vi "AO_mini_AndorEMCCD.vi"() -> ()   [LabVIEW 2018]
panel:
  in  "Auto Scale":bool=TRUE caption="PD Correction"
  out "Get EMCCD Gain":i32=1
  in  "Spool":bool=TRUE caption="Cameras Live Display"
  out "Return from SetSpool":i32=1
  out "Running Status":T1(ring) caption="Camera FOV"
  out "Return from Start Acquisition":u32
  out "Return from GetAcquiredData":u32
  in  "Folder Name":string="test"
  in  "File Type":enum16{"TIFF", "Sif"}(ring)
  out "Return from CheckProcess":u32
  out "Get Kinetic Time":sgl format="%.4f"
  out "Get Accum Time":sgl format="%.4f"
  out "Get Kinetic Num":i32=1
  out "Get Accum Num":i32=1
  in  "Abort":bool
  out "FOV Y Pixels":i32
  out "FOV X Pixels":i32
  in  "Acquisition":bool
  in  "Exit":bool
  out "EMCCD Status":bool
  in  "Stop LIVE":bool
  in  "Start LIVE":bool
  out "error out":errorcluster
  out "Return from CheckTimings":u32
  out "Get Exposure Time":sgl format="%.4f"
  in  "error in (no error)":errorcluster
  in  "Intensity Min":dbl=200.0 min=1.0
  in  "Intensity Max":dbl=10000.0 min=1.0
  in  "Shutdown EMCCD when exit":bool=TRUE caption="PD Correction"
  in  "Update FOV":bool
  in  "Update AcqSetting":bool
  in  "Exposure time (s)":dbl=0.02
  in  "Main Path":path=path "D:/Data"
  in  "File Name":string="test"
  in  "Kinetic Num":u32=5
  in  "Accum Num":u32=2
  in  "Initialize EMCCD":bool=TRUE caption="PD Correction"
  in  "CoolToTargetTemp":bool=TRUE caption="PD Correction"
  out "Intensity Graph":i32[][](graph)
  out "Current Temp":i32
  out "Detector Y Pixels":i32
  out "Detector X Pixels":i32
  in  "Aquisition Mode":T2(ring)=enum."Single Scan" caption="Camera FOV"
  in  "Trigger Mode":enum16{"Internal", "External"}(ring) caption="Camera FOV"
  in  "Gain Value":sgl=20.0 format="%.2f"
  in  "Yend":i32=1002
  in  "Xend":i32=1004
  in  "Ystart":i32=2
  in  "Xstart":i32=2
  in  "Ybin":i32=1
  in  "Xbin":i32=1
  in  "Camera FOV":T3(ring)=enum."Full FOV"
  in  "Gain On":bool=TRUE caption="Cameras Live Display"
  in  "Set Temp":i32=-60
  # "It takes some time to warm up / cool down the camera when initializing or shuting down the camera (without Temp feedback)"
  # "C"
  # "Acquisition Settings"
  # "Status"
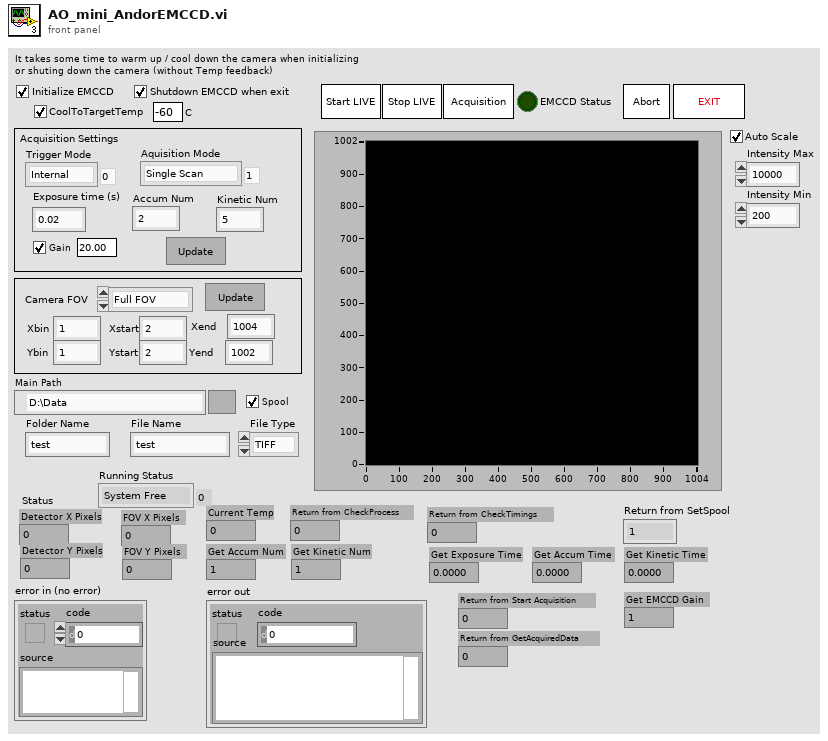
[diagram p1: front panel]
types:
  T1 = enum16{"System Free", "Live Preview", "Data Acquisition"}
  T2 = enum16{"None", "Single Scan", "Accumulate", "Kinetics", "Fast Kinetics", "Run till abort"}
  T3 = enum16{"Custom FOV", "Full FOV", "FOV: 768x768", "FOV: 512x512", "FOV: 320x320", "FOV: 256x256", ""}
  T4 = typedef "Error Code Enum typedef.ctl" = enum32{"N/A (0)", "DRV_ERROR_CODES", "DRV_SUCCESS", "DRV_VXDNOTINSTALLED", "DRV_ERROR_SCAN", "DRV_ERROR_CHECK_SUM", "DRV_ERROR_FILELOAD", "DRV_UNKNOWN_FUNC", "DRV_ERROR_VXD_INIT", "DRV_ERROR_ADDRESS", "DRV_ERROR_PAGELOCK", "DRV_ERROR_PAGEUNLOCK", "DRV_ERROR_BOARDTEST", "DRV_ERROR_ACK", "DRV_ERROR_UP_FIFO", "DRV_ERROR_PATTERN", "N/A (16)", "DRV_ACQUISITION_ERRORS", "DRV_ACQ_BUFFER", "DRV_ACQ_DOWNFIFO_FULL", "DRV_PROC_UNKONWN_INSTRUCTION", "DRV_ILLEGAL_OP_CODE", "DRV_KINETIC_TIME_NOT_MET", "DRV_ACCUM_TIME_NOT_MET", "DRV_NO_NEW_DATA", "N/A (25)", "DRV_SPOOLERROR", "N/A (27)", "N/A (28)", "N/A (29)", "N/A (30)", "N/A (31)", "N/A (32)", "DRV_TEMPERATURE_CODES", "DRV_TEMPERATURE_OFF", "DRV_TEMPERATURE_NOT_STABILIZED", "DRV_TEMPERATURE_STABILIZED", "DRV_TEMPERATURE_NOT_REACHED", "DRV_TEMPERATURE_OUT_RANGE", "DRV_TEMPERATURE_NOT_SUPPORTED", "DRV_TEMPERATURE_DRIFT", "N/A (41)", "N/A (42)", "N/A (43)", "N/A (44)", "N/A (45)", "N/A (46)", "N/A (47)", "N/A (48)", "DRV_GENERAL_ERRORS", "DRV_INVALID_AUX", "DRV_COF_NOTLOADED", "DRV_FPGAPROG", "DRV_FLEXERROR", "DRV_GPIBERROR", "N/A (55)", "N/A (56)", "N/A (57)", "N/A (58)", "N/A (59)", "N/A (60)", "N/A (61)", "N/A (62)", "N/A (63)", "DRV_DATATYPE", "DRV_DRIVER_ERRORS", "DRV_P1INVALID", "DRV_P2INVALID", "DRV_P3INVALID", "DRV_P4INVALID", "DRV_INIERROR", "DRV_COFERROR", "DRV_ACQUIRING", "DRV_IDLE", "DRV_TEMPCYCLE", "DRV_NOT_INITIALIZED", "DRV_P5INVALID", "DRV_P6INVALID", "DRV_INVALID_MODE", "DRV_INVALID_FILTER", "DRV_I2CERRORS", "DRV_I2CDEVNOTFOUND", "DRV_I2CTIMEOUT", "DRV_P7INVALID", "N/A (84)", "N/A (85)", "N/A (86)", "N/A (87)", "N/A (88)", "N/A (89)", "DRV_IOCERROR", "DRV_VRMVERSIONERROR"}
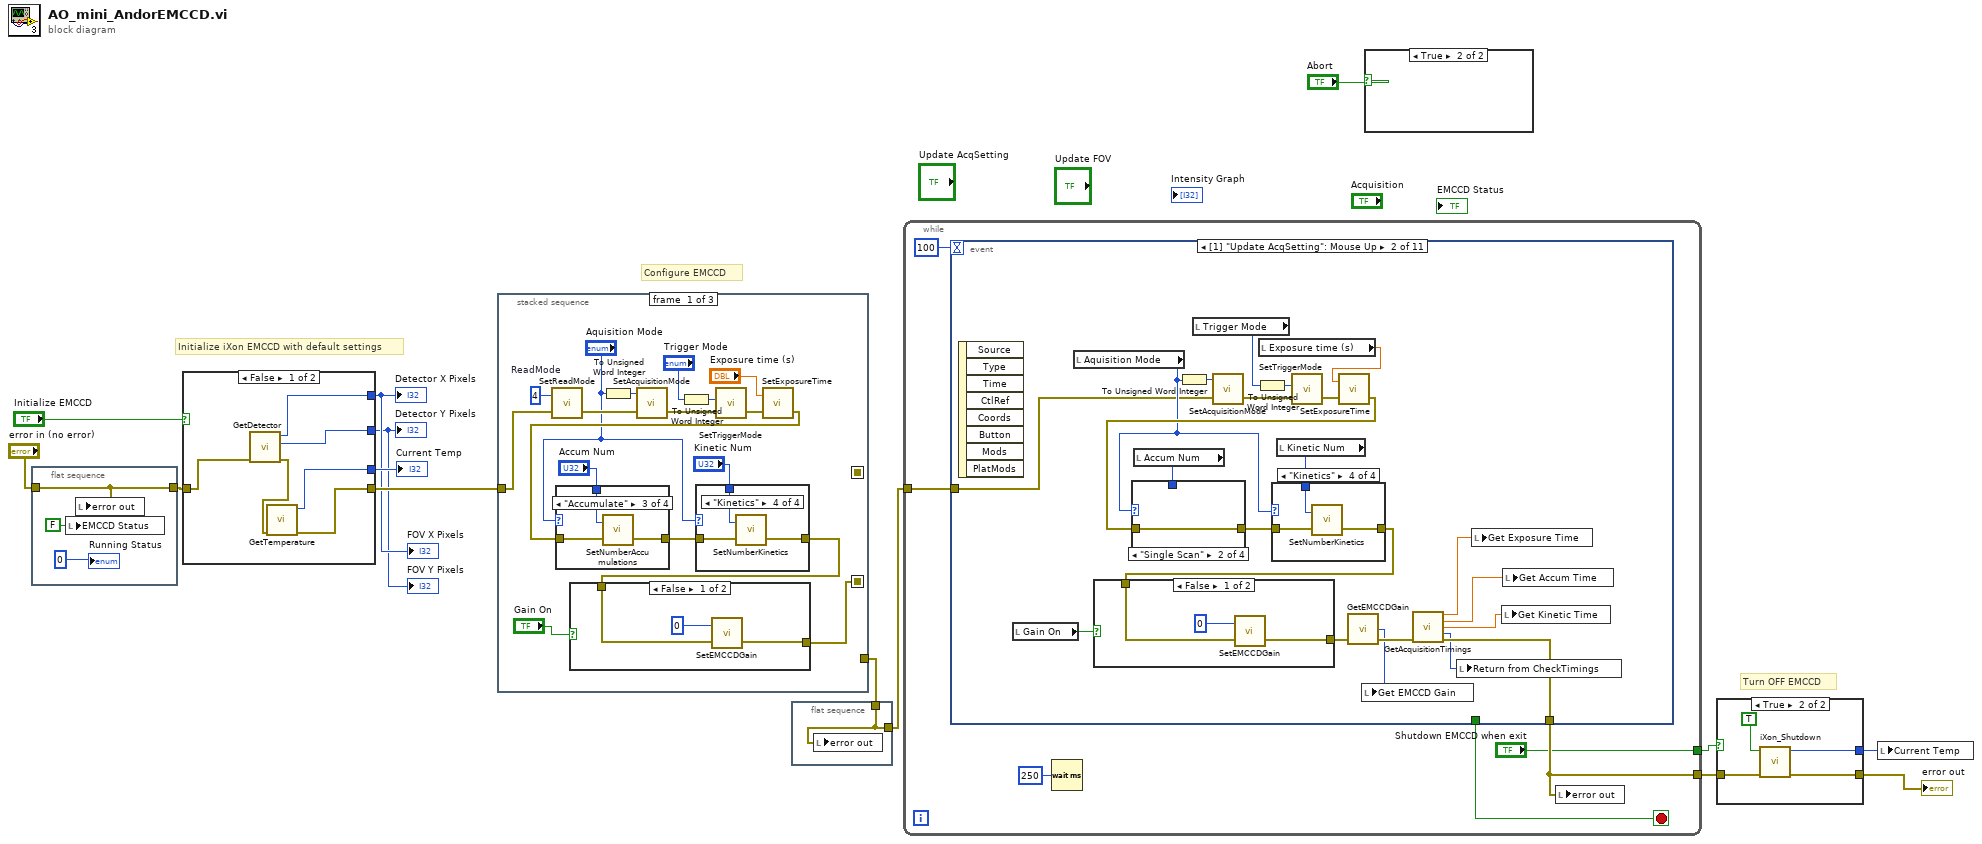
[diagram p0: block diagram]
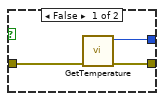
[diagram p3: hidden frame]
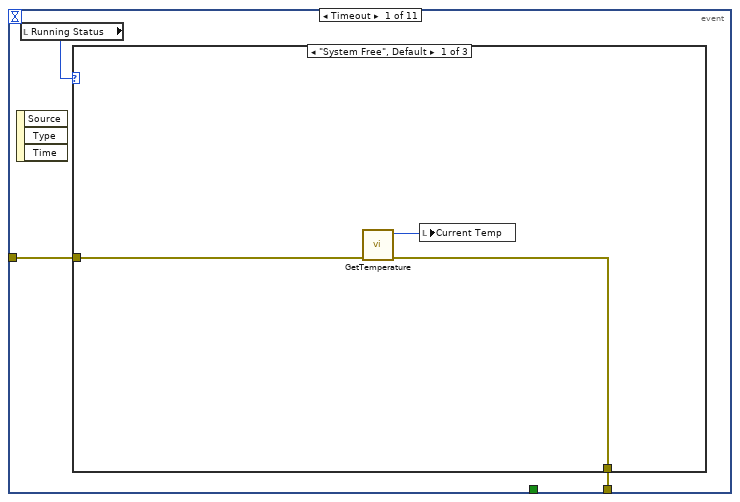
[diagram p4: hidden frame]
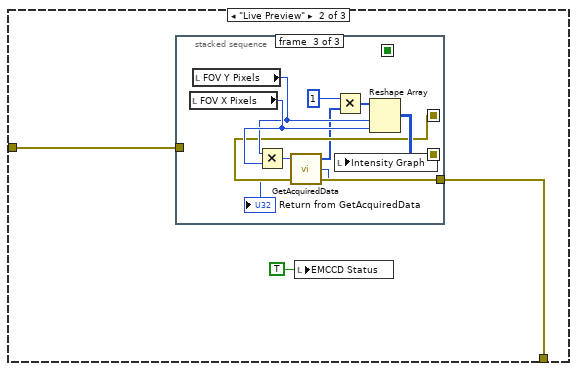
[diagram p5: hidden frame]
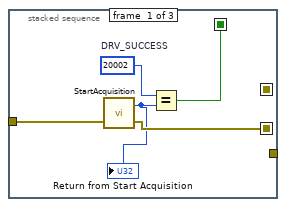
[diagram p6: hidden frame]
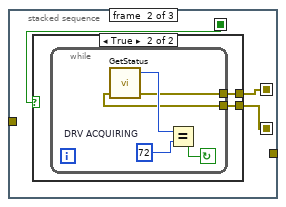
[diagram p7: hidden frame]
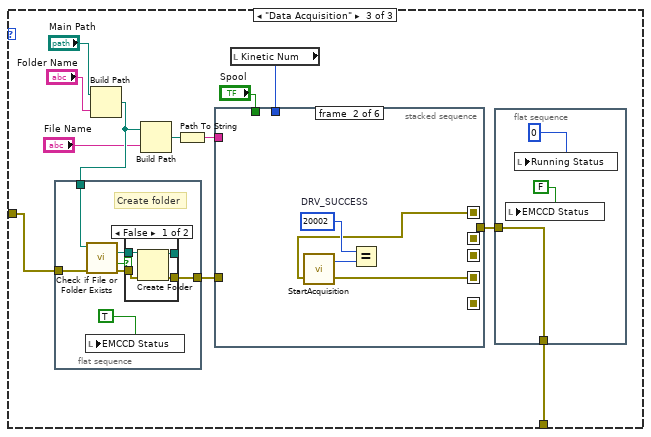
[diagram p9: hidden frame]
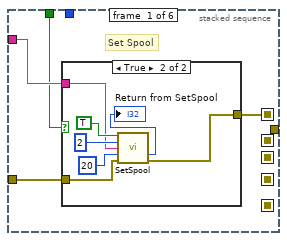
[diagram p10: hidden frame]
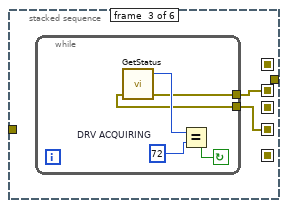
[diagram p12: hidden frame]
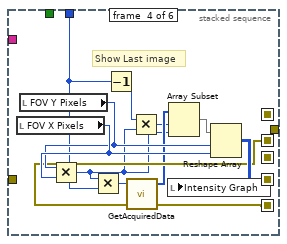
[diagram p13: hidden frame]
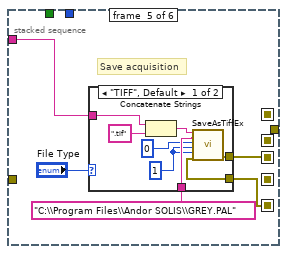
[diagram p14: hidden frame]
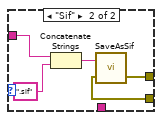
[diagram p15: hidden frame]
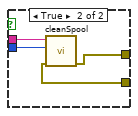
[diagram p17: hidden frame]
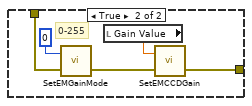
[diagram p19: hidden frame]
diagram:
  # "Turn OFF EMCCD"
  # "Configure EMCCD"
  # "Initialize iXon EMCCD with default settings"
  n1 = flat-sequence {
    tunnel: "error in (no error)" -> [w17]
    tunnel: [w17] -> w5
    frame #0 {
      n2 = local write "EMCCD Status"(FALSE) -> ()
      n3 = local write "error out"(w17) -> ()
      "Running Status" <- u16 0
    }
  }
  n4 = case shown="False" "Initialize EMCCD" {
    tunnel: w5 -> [w22 w29]
    tunnel: [w20 w27] -> w11
    tunnel: [w19 w26] -> w10
    tunnel: [w23 w25] -> w13
    tunnel: [w18 w24] -> w12
    frame False {
      n5 = call <userlib>:"GetDetector.vi"("error in (no error)"=w22) -> ("error out"=w21:errorcluster, "ypixels"=w19:i32, "xpixels"=w20:i32)  [unwired: 3 in, 1 out]
      n6 = call <userlib>:"GetTemperature.vi"("error in (no error)"=w21) -> ("error out"=w18:errorcluster, "temperature"=w23:i32)  [unwired: 3 in, 2 out]
    }
    frame True {
      n7 = call "iXon_Init_Cool.vi"("error in (no error)"=w29, "CoolToTargetTemp"="CoolToTargetTemp", "Set Temp"="Set Temp") -> ("error out"=w24:errorcluster, "Current Temp"=w25:i32, "Detector Y Pixels"=w26:i32, "Detector X Pixels"=w27:i32)  [unwired: 5 in]
    }
  }
  "Detector X Pixels" <- w11
  "Detector Y Pixels" <- w10
  "Current Temp" <- w13
  "FOV X Pixels" <- w11
  "FOV Y Pixels" <- w10
  n8 = stacked-sequence {
    seq-local: [w31 _ _] -> [_ w75 _]
    seq-local: [_ w74 _] -> [_ _ w173]
    tunnel: w12 -> [w45 _ _]
    tunnel: [_ _ w165] -> w4
    frame #0 {
      w46 = u16 4  # ReadMode
      n9 = call <userlib>:"SetReadMode.vi"("error in (no error)"=w45, "mode"=w46) -> ("error out"=w43:errorcluster)  [unwired: 1 out]
      n10 = To Unsigned Word Integer(number="Aquisition Mode") -> (unsigned 16bit integer=w47:u16)
      n11 = call <userlib>:"SetAcquisitionMode.vi"("error in (no error)"=w43, "mode"=w47) -> ("error out"=w42:errorcluster)  [unwired: 1 out]
      n12 = To Unsigned Word Integer(number="Trigger Mode") -> (unsigned 16bit integer=w41:u16)
      n13 = call <userlib>:"SetTriggerMode.vi"("error in (no error)"=w42, "mode"=w41) -> ("error out"=w40:errorcluster)  [unwired: 1 out]
      n14 = call <userlib>:"SetExposureTime.vi"("error in (no error)"=w40, "time"="Exposure time (s)") -> ("error out"=w37:errorcluster)  [unwired: 1 out]
      n15 = case shown="\"Accumulate\"" "Aquisition Mode" {
        tunnel: "Accum Num" -> [_ _ w66 w69]
        tunnel: w37 -> [w62 w63 w65 w68]
        tunnel: [w62 w63 w64 w67] -> w36
        frame "None", Default {
        }
        frame "Single Scan" {
        }
        frame "Accumulate" {
          n16 = call <userlib>:"SetNumberAccumulations.vi"("error in (no error)"=w65, "number"=w66) -> ("error out"=w64:errorcluster)  [unwired: 1 out]
        }
        frame "Kinetics" {
          n17 = call <userlib>:"SetNumberAccumulations.vi"("error in (no error)"=w68, "number"=w69) -> ("error out"=w67:errorcluster)  [unwired: 1 out]
        }
      }
      n18 = case shown="\"Kinetics\"" "Aquisition Mode" {
        tunnel: w36 -> [w56 w57 w58 w61]
        tunnel: [w56 w57 w58 w60] -> w32
        tunnel: "Kinetic Num" -> [_ _ _ w59]
        frame "None", Default {
        }
        frame "Single Scan" {
        }
        frame "Accumulate" {
        }
        frame "Kinetics" {
          n19 = call <userlib>:"SetNumberKinetics.vi"("error in (no error)"=w61, "number"=w59) -> ("error out"=w60:errorcluster)  [unwired: 1 out]
        }
      }
      n20 = case shown="False" "Gain On" {
        tunnel: w32 -> [w50 w55]
        tunnel: [w49 w52] -> w31
        frame False {
          n21 = call <userlib>:"SetEMCCDGain.vi"("error in (no error)"=w50, "gain"=u16 0) -> ("error out"=w49:errorcluster)  [unwired: 1 out]
        }
        frame True {
          # "0-255"
          n22 = call <userlib>:"SetEMGainMode.vi"("error in (no error)"=w55, "mode"=0) -> ("error out"=w53:errorcluster)  [unwired: 1 out]
          n23 = call <userlib>:"SetEMCCDGain.vi"("error in (no error)"=w53, "gain"="Gain Value") -> ("error out"=w52:errorcluster)  [unwired: 1 out]
        }
      }
    }
    frame #1 {
      # "Set FOV"
      n24 = local read "Detector X Pixels"() -> (w73:i32)
      n25 = local read "Detector Y Pixels"() -> (w72:i32)
      n26 = case shown="\"Custom FOV\"" "Camera FOV" {
        tunnel: ["Xbin" w112 w128 w144 w160 w163] -> w81
        tunnel: ["Ybin" w112 w128 w144 w160 w163] -> w80
        tunnel: ["Xstart" w102 w118 w134 w150 w163] -> w79
        tunnel: ["Xend" w99 w115 w131 w147 w161] -> w78
        tunnel: ["Ystart" w101 w117 w133 w149 w163] -> w77
        tunnel: ["Yend" w98 w114 w130 w146 w162] -> w76
        tunnel: w73 -> [_ w111 w127 w143 w159 w161]
        tunnel: w72 -> [_ w110 w126 w142 w158 w162]
        tunnel: [w83 w97 w113 w129 w145 w162] -> w71
        tunnel: [w86 w97 w113 w129 w145 w161] -> w70
        frame "Custom FOV" {
          n27 = Subtract(x="Yend", y="Ystart") -> (x-y=w93:i32)
          n28 = Subtract(x="Xend", y="Xstart") -> (x-y=w96:i32)
          n29 = Increment(x=w93) -> (x+1=w90:i32)
          n30 = Increment(x=w96) -> (x+1=w89:i32)
          n31 = Divide(x=w90, y="Ybin") -> (x/y=w84:dbl)
          n32 = Divide(x=w89, y="Xbin") -> (x/y=w87:dbl)
          n33 = To Long Integer(number=w84) -> (32bit integer=w83:i32)
          n34 = To Long Integer(number=w87) -> (32bit integer=w86:i32)
        }
        frame "FOV: 768x768" {
          w97 = 768
          w107 = 2.0
          w112 = 1
          n35 = Subtract(x=w111, y=w97) -> (x-y=w109:i32)
          n36 = Subtract(x=w110, y=w97) -> (x-y=w108:i32)
          n37 = Divide(x=w108, y=w107) -> (x/y=w105:dbl)
          n38 = Divide(x=w109, y=w107) -> (x/y=w106:dbl)
          n39 = Decrement(x=w97) -> (x-1=w100:i32)
          n40 = Round To Nearest(number=w106) -> (nearest integer value=w104:dbl)
          n41 = Round To Nearest(number=w105) -> (nearest integer value=w103:dbl)
          n42 = To Long Integer(number=w104) -> (32bit integer=w102:i32)
          n43 = To Long Integer(number=w103) -> (32bit integer=w101:i32)
          n44 = Add(x=w100, y=w102) -> (x+y=w99:i32)
          n45 = Add(x=w100, y=w101) -> (x+y=w98:i32)
        }
        frame "FOV: 512x512" {
          w113 = 512
          w123 = 2.0
          w128 = 1
          n46 = Subtract(x=w127, y=w113) -> (x-y=w125:i32)
          n47 = Subtract(x=w126, y=w113) -> (x-y=w124:i32)
          n48 = Divide(x=w124, y=w123) -> (x/y=w121:dbl)
          n49 = Divide(x=w125, y=w123) -> (x/y=w122:dbl)
          n50 = Decrement(x=w113) -> (x-1=w116:i32)
          n51 = Round To Nearest(number=w122) -> (nearest integer value=w120:dbl)
          n52 = Round To Nearest(number=w121) -> (nearest integer value=w119:dbl)
          n53 = To Long Integer(number=w120) -> (32bit integer=w118:i32)
          n54 = To Long Integer(number=w119) -> (32bit integer=w117:i32)
          n55 = Add(x=w116, y=w118) -> (x+y=w115:i32)
          n56 = Add(x=w116, y=w117) -> (x+y=w114:i32)
        }
        frame "FOV: 320x320" {
          w129 = 320
          w139 = 2.0
          w144 = 1
          n57 = Subtract(x=w143, y=w129) -> (x-y=w141:i32)
          n58 = Subtract(x=w142, y=w129) -> (x-y=w140:i32)
          n59 = Divide(x=w140, y=w139) -> (x/y=w137:dbl)
          n60 = Divide(x=w141, y=w139) -> (x/y=w138:dbl)
          n61 = Decrement(x=w129) -> (x-1=w132:i32)
          n62 = Round To Nearest(number=w138) -> (nearest integer value=w136:dbl)
          n63 = Round To Nearest(number=w137) -> (nearest integer value=w135:dbl)
          n64 = To Long Integer(number=w136) -> (32bit integer=w134:i32)
          n65 = To Long Integer(number=w135) -> (32bit integer=w133:i32)
          n66 = Add(x=w132, y=w134) -> (x+y=w131:i32)
          n67 = Add(x=w132, y=w133) -> (x+y=w130:i32)
        }
        frame "FOV: 256x256" {
          w145 = 256
          w155 = 2.0
          w160 = 1
          n68 = Subtract(x=w159, y=w145) -> (x-y=w157:i32)
          n69 = Subtract(x=w158, y=w145) -> (x-y=w156:i32)
          n70 = Divide(x=w156, y=w155) -> (x/y=w153:dbl)
          n71 = Divide(x=w157, y=w155) -> (x/y=w154:dbl)
          n72 = Decrement(x=w145) -> (x-1=w148:i32)
          n73 = Round To Nearest(number=w154) -> (nearest integer value=w152:dbl)
          n74 = Round To Nearest(number=w153) -> (nearest integer value=w151:dbl)
          n75 = To Long Integer(number=w152) -> (32bit integer=w150:i32)
          n76 = To Long Integer(number=w151) -> (32bit integer=w149:i32)
          n77 = Add(x=w148, y=w150) -> (x+y=w147:i32)
          n78 = Add(x=w148, y=w149) -> (x+y=w146:i32)
        }
        frame "Full FOV", Default {
          w163 = 1
        }
      }
      n79 = local write "FOV X Pixels"(w70) -> ()
      n80 = local write "FOV Y Pixels"(w71) -> ()
      n81 = call <userlib>:"SetImage.vi"("hbin"=w81, "vbin"=w80, "hstart"=w79, "hend"=w78, "vstart"=w77, "vend"=w76, "error in (no error)"=w75) -> ("error out"=w74:errorcluster)  [unwired: 19 in, 1 out]
    }
    frame #2 {
      n82 = call <userlib>:"GetAcquisitionTimings.vi"("error in (no error)"=w173) -> ("exposure"=→"Get Exposure Time":sgl, "accumulate"=→"Get Accum Time":sgl, "kinetic"=→"Get Kinetic Time":sgl, "DLL error code"=→"Return from CheckTimings":u32, "error out"=w172:errorcluster)  [unwired: 10 in]
      n83 = call <userlib>:"GetAcquisitionProgress.vi"("error in (no error)"=w172) -> ("error out"=w166:errorcluster, "DLL error code"=→"Return from CheckProcess":u32, "series"=→"Get Kinetic Num":i32, "accum"=→"Get Accum Num":i32)  [unwired: 3 in]
      n84 = call <userlib>:"GetEMCCDGain.vi"("error in (no error)"=w166) -> ("error out"=w165:errorcluster, "gain"=→"Get EMCCD Gain":u32)  [unwired: 2 in, 1 out]
    }
  }
  n85 = flat-sequence {
    tunnel: w4 -> [w176]
    tunnel: [w176] -> w3
    frame #0 {
      n86 = local write "error out"(w176) -> ()
    }
  }
  n87 = while {
    tunnel: w3 -> [w181]
    tunnel: [w179] -> w9
    tunnel: ["Shutdown EMCCD when exit"] -> w2
    stop <- w180 stop-if-true
    n88 = event shown="[1] \"Update AcqSetting\": Mouse Up" {
      selector: _ -> [_ _ _ _ _ _ _ _ _ _ _]
      dyn-events: _ -> [_ _ _ _ _ _ _ _ _ _ _]
      timeout: 100 -> [_ _ _ _ _ _ _ _ _ _ _]
      tunnel: w181 -> [w183 w319 w363 w458 w467 w476 w479 _ _ w481 w484]
      tunnel: [w184 w317 w360 w457 w465 w476 w478 _ _ w481 w484] -> w179
      tunnel: [_ _ _ _ _ _ _ _ _ TRUE ("Exit") TRUE ("Exit")] -> w180
      event Timeout {
        n89 = event-data() -> ()  [unwired: 1 in, 3 out]
        n90 = local read "Running Status"() -> (w185:T1)
        n91 = case shown="\"System Free\", Default" w185 {
          tunnel: [w186 w191 w225] -> w184
          tunnel: w183 -> [w187 w190 w224]
          frame "System Free", Default {
            n92 = call <userlib>:"GetTemperature.vi"("error in (no error)"=w187) -> ("error out"=w186:errorcluster, "temperature"=w188:i32)  [unwired: 3 in, 2 out]
            n93 = local write "Current Temp"(w188) -> ()
          }
          frame "Live Preview" {
            n94 = stacked-sequence {
              seq-local: [w194 _ _] -> [_ w199 _]
              seq-local: [_ w198 _] -> [_ _ w213]
              seq-local: [w193 _ _] -> [_ w197 _]
              tunnel: w190 -> [w195 _ _]
              tunnel: [_ _ w212] -> w191
              frame #0 {
                w196 = 20002  # DRV_SUCCESS
                n95 = call <userlib>:"StartAcquisition.vi"("error in (no error)"=w195) -> ("error out"=w194:errorcluster, "DLL error code"=w192:u32)  [unwired: 1 in]
                "Return from Start Acquisition" <- w192
                n96 = Equal?(x=w196, y=w192) -> (x = y?=w193:bool)
              }
              frame #1 {
                n97 = case shown="True" w197 {
                  tunnel: w199 -> [w200 w202]
                  tunnel: [w200 w201] -> w198
                  frame False {
                  }
                  frame True {
                    n98 = while {
                      tunnel: w202 -> [w204]
                      tunnel: [w203] -> w201
                      stop <- w205 continue-if-true
                      w207 = u16 72  # DRV ACQUIRING
                      n99 = call <userlib>:"GetStatus.vi"("error in (no error)"=w204) -> ("error out"=w203:errorcluster, "status"=w206:T4)  [unwired: 2 in, 1 out]
                      n100 = Equal?(x=w206, y=w207) -> (x = y?=w205:bool)
                    }
                  }
                }
              }
              frame #2 {
                n101 = local read "FOV X Pixels"() -> (w216:i32)
                n102 = local read "FOV Y Pixels"() -> (w215:i32)
                n103 = Multiply(x=w215, y=w216) -> (x*y=w217:i32)
                n104 = call <userlib>:"GetAcquiredData.vi"("error in (no error)"=w213, "size"=w217) -> ("error out"=w212:errorcluster, "DLL error code"=→"Return from GetAcquiredData":u32, "array"=w208:i32[])  [unwired: 1 in]
                n105 = Multiply(x=1, y=w208) -> (x*y=w209:i32[])
                n106 = Reshape Array(w209, w215, w216) -> (w214:i32[][])
                n107 = local write "Intensity Graph"(w214) -> ()
              }
            }
            n108 = local write "EMCCD Status"(TRUE) -> ()
          }
          frame "Data Acquisition" {
            n109 = flat-sequence {
              tunnel: [w296] -> w229
              tunnel: w224 -> [w298]
              tunnel: w226 -> [w299]
              frame #0 {
                # "Create folder"
                n110 = local write "EMCCD Status"(TRUE) -> ()
                n111 = call <vilib>:"Check if File or Folder Exists.vi"("error in (no error)"=w298, "path"=w299) -> ("error out"=w297:errorcluster, "file or folder exists?"=w301:bool, "dup path"=w300:path)  [unwired: 7 in]
                n112 = case shown="False" w301 {
                  tunnel: w300 -> [w306 w308]
                  tunnel: [w305 w308] -> _
                  tunnel: w297 -> [w304 w307]
                  tunnel: [w303 w307] -> w296
                  frame False {
                    n113 = Create Folder(path (use dialog)=w306, error in=w304) -> (created path=w305:path, error out=w303:errorcluster)  [unwired: 1 in, 1 out]
                  }
                  frame True {
                  }
                }
              }
            }
            n114 = Build Path(base path="Main Path", name or relative path="Folder Name") -> (appended path=w226:path)
            n115 = Build Path(base path=w226, name or relative path="File Name") -> (appended path=w222:path)
            n116 = Path To String(path=w222) -> (string=w221:string)
            n117 = local read "Kinetic Num"() -> (w220:u32)
            n118 = stacked-sequence {
              seq-local: [_ w243 _ _ _ _] -> [_ _ w247 _ _ _]
              seq-local: [_ _ w246 _ _ _] -> [_ _ _ w261 _ _]
              seq-local: [_ _ _ w256 _ _] -> [_ _ _ _ w267 _]
              seq-local: [w231 _ _ _ _ _] -> [_ w242 _ _ _ _]
              seq-local: [_ _ _ _ w265 _] -> [_ _ _ _ _ w286]
              tunnel: w229 -> [w232 _ _ _ _ _]
              tunnel: w221 -> [w233 _ _ _ w266 w284]
              tunnel: w220 -> [_ _ _ w253 _ w287]
              tunnel: "Spool" -> [w230 _ _ _ _ w283]
              tunnel: [_ _ _ _ _ w285] -> w218
              frame #0 {
                # "Set Spool"
                n119 = case shown="True" w230 {
                  tunnel: w233 -> [_ w238]
                  tunnel: w232 -> [w234 w237]
                  tunnel: [w234 w235] -> w231
                  frame False {
                  }
                  frame True {
                    n120 = call <userlib>:"SetSpool.vi"("active"=TRUE, "method"=2, "name"=w238, "framebuffersize (10)"=20, "error in (no error)"=w237) -> ("DLL error code"=→"Return from SetSpool":u32, "error out"=w235:errorcluster)  [unwired: 9 in]
                  }
                }
              }
              frame #1 {
                w244 = 20002  # DRV_SUCCESS
                n121 = call <userlib>:"StartAcquisition.vi"("error in (no error)"=w242) -> ("error out"=w243:errorcluster, "DLL error code"=w245:u32)  [unwired: 1 in]
                n122 = Equal?(x=w244, y=w245) -> ()  [unwired: 1 out]
              }
              frame #2 {
                n123 = while {
                  tunnel: w247 -> [w249]
                  tunnel: [w248] -> w246
                  stop <- w250 continue-if-true
                  w252 = u16 72  # DRV ACQUIRING
                  n124 = call <userlib>:"GetStatus.vi"("error in (no error)"=w249) -> ("error out"=w248:errorcluster, "status"=w251:T4)  [unwired: 2 in, 1 out]
                  n125 = Equal?(x=w251, y=w252) -> (x = y?=w250:bool)
                }
              }
              frame #3 {
                # "Show Last image"
                n126 = local read "FOV X Pixels"() -> (w264:i32)
                n127 = local read "FOV Y Pixels"() -> (w263:i32)
                n128 = Multiply(x=w263, y=w264) -> (x*y=w254:i32)
                n129 = Multiply(x=w254, y=w253) -> (x*y=w255:u32)
                n130 = Decrement(x=w253) -> (x-1=w257:u32)
                n131 = call <userlib>:"GetAcquiredData.vi"("error in (no error)"=w261, "size"=w255) -> ("error out"=w256:errorcluster, "array"=w260:i32[])  [unwired: 1 in, 1 out]
                n132 = Multiply(x=w257, y=w254) -> (x*y=w258:u32)
                n133 = Array Subset(array=w260, index=w258, length=w254) -> (w259:i32[])
                n134 = Reshape Array(w259, w263, w264) -> (w262:i32[][])
                n135 = local write "Intensity Graph"(w262) -> ()
              }
              frame #4 {
                # "Save acquisition"
                n136 = case shown="\"TIFF\", Default" "File Type" {
                  tunnel: "C:\\Program Files\\Andor SOLIS\\GREY.PAL" -> [w273 _]
                  tunnel: w266 -> [w276 w282]
                  tunnel: w267 -> [w274 w279]
                  tunnel: [w275 w278] -> w265
                  frame "TIFF", Default {
                    w270 = 1
                    n137 = Concatenate Strings(w276, ".tif") -> (w272:string)
                    n138 = call <userlib>:"SaveAsTiffEx.vi"("path"=w272, "palette"=w273, "position"=0, "type"=w270, "mode"=w270, "error in (no error)"=w274) -> ("error out"=w275:errorcluster)  [unwired: 12 in, 1 out]
                  }
                  frame "Sif" {
                    n139 = Concatenate Strings(w282, ".sif") -> (w280:string)
                    n140 = call <userlib>:"SaveAsSif.vi"("error in (no error)"=w279, "path"=w280) -> ("error out"=w278:errorcluster)  [unwired: 1 out]
                  }
                }
              }
              frame #5 {
                # "Clearn Spool Files"
                n141 = case shown="False" w283 {
                  tunnel: w287 -> [_ w292]
                  tunnel: w286 -> [w288 w291]
                  tunnel: [w288 w290] -> w285
                  tunnel: w284 -> [_ w289]
                  frame False {
                  }
                  frame True {
                    n142 = call "cleanSpool.vi"("error in (no error)"=w291, "Total Img Num"=w292, "strPath"=w289) -> ("error out"=w290:errorcluster)  [unwired: 8 in]
                  }
                }
              }
            }
            n143 = flat-sequence {
              tunnel: w218 -> [w294]
              tunnel: [w294] -> w225
              frame #0 {
                n144 = local write "EMCCD Status"(FALSE) -> ()
                n145 = local write "Running Status"(0) -> ()
              }
            }
          }
        }
      }
      event "Update AcqSetting": Mouse Up {
        n146 = event-data() -> ()  [unwired: 1 in, 8 out]
        n147 = local read "Gain On"() -> (w310:bool)
        n148 = local read "Aquisition Mode"() -> (w322:T2)
        n149 = local read "Accum Num"() -> (w324:u32)
        n150 = To Unsigned Word Integer(number=w322) -> (unsigned 16bit integer=w330:u16)
        n151 = local read "Trigger Mode"() -> (w321:enum16{"Internal", "External"})
        n152 = call <userlib>:"SetAcquisitionMode.vi"("error in (no error)"=w319, "mode"=w330) -> ("error out"=w329:errorcluster)  [unwired: 1 out]
        n153 = To Unsigned Word Integer(number=w321) -> (unsigned 16bit integer=w328:u16)
        n154 = local read "Exposure time (s)"() -> (w320:dbl)
        n155 = local read "Kinetic Num"() -> (w323:u32)
        n156 = call <userlib>:"SetTriggerMode.vi"("error in (no error)"=w329, "mode"=w328) -> ("error out"=w327:errorcluster)  [unwired: 1 out]
        n157 = call <userlib>:"SetExposureTime.vi"("error in (no error)"=w327, "time"=w320) -> ("error out"=w326:errorcluster)  [unwired: 1 out]
        n158 = case shown="\"Single Scan\"" w322 {
          tunnel: w324 -> [_ _ w349 w352]
          tunnel: w326 -> [w345 w346 w348 w351]
          tunnel: [w345 w346 w347 w350] -> w325
          frame "None", Default {
          }
          frame "Single Scan" {
          }
          frame "Accumulate" {
            n159 = call <userlib>:"SetNumberAccumulations.vi"("error in (no error)"=w348, "number"=w349) -> ("error out"=w347:errorcluster)  [unwired: 1 out]
          }
          frame "Kinetics" {
            n160 = call <userlib>:"SetNumberAccumulations.vi"("error in (no error)"=w351, "number"=w352) -> ("error out"=w350:errorcluster)  [unwired: 1 out]
          }
        }
        n161 = case shown="\"Kinetics\"" w322 {
          tunnel: w325 -> [w339 w340 w341 w344]
          tunnel: [w339 w340 w341 w343] -> w311
          tunnel: w323 -> [_ _ _ w342]
          frame "None", Default {
          }
          frame "Single Scan" {
          }
          frame "Accumulate" {
          }
          frame "Kinetics" {
            n162 = call <userlib>:"SetNumberKinetics.vi"("error in (no error)"=w344, "number"=w342) -> ("error out"=w343:errorcluster)  [unwired: 1 out]
          }
        }
        n163 = case shown="False" w310 {
          tunnel: w311 -> [w331 w338]
          tunnel: [w332 w335] -> w309
          frame False {
            n164 = call <userlib>:"SetEMCCDGain.vi"("error in (no error)"=w331, "gain"=u16 0) -> ("error out"=w332:errorcluster)  [unwired: 1 out]
          }
          frame True {
            # "0-255"
            n165 = call <userlib>:"SetEMGainMode.vi"("error in (no error)"=w338, "mode"=0) -> ("error out"=w336:errorcluster)  [unwired: 1 out]
            n166 = local read "Gain Value"() -> (w334:sgl)
            n167 = call <userlib>:"SetEMCCDGain.vi"("error in (no error)"=w336, "gain"=w334) -> ("error out"=w335:errorcluster)  [unwired: 1 out]
          }
        }
        n168 = call <userlib>:"GetEMCCDGain.vi"("error in (no error)"=w309) -> ("error out"=w313:errorcluster, "gain"=w312:u32)  [unwired: 2 in, 1 out]
        n169 = local write "Get EMCCD Gain"(w312) -> ()
        n170 = call <userlib>:"GetAcquisitionTimings.vi"("error in (no error)"=w313) -> ("exposure"=w318:sgl, "accumulate"=w315:sgl, "kinetic"=w314:sgl, "DLL error code"=w316:u32, "error out"=w317:errorcluster)  [unwired: 10 in]
        n171 = local write "Return from CheckTimings"(w316) -> ()
        n172 = local write "Get Exposure Time"(w318) -> ()
        n173 = local write "Get Kinetic Time"(w314) -> ()
        n174 = local write "Get Accum Time"(w315) -> ()
      }
      event "Update FOV": Value Change {
        n175 = event-data() -> ()  [unwired: 1 in, 6 out]
        n176 = local read "Detector Y Pixels"() -> (w373:i32)
        n177 = local read "Detector X Pixels"() -> (w374:i32)
        n178 = local read "Camera FOV"() -> (w372:T3)
        n179 = case shown="\"Custom FOV\"" w372 {
          tunnel: [w380 w404 w420 w436 w452 w455] -> w368
          tunnel: [w379 w404 w420 w436 w452 w455] -> w369
          tunnel: [w378 w394 w410 w426 w442 w455] -> w370
          tunnel: [w377 w391 w407 w423 w439 w453] -> w371
          tunnel: [w375 w393 w409 w425 w441 w455] -> w367
          tunnel: [w376 w390 w406 w422 w438 w454] -> w366
          tunnel: w374 -> [_ w403 w419 w435 w451 w453]
          tunnel: w373 -> [_ w402 w418 w434 w450 w454]
          tunnel: [w381 w389 w405 w421 w437 w454] -> w364
          tunnel: [w383 w389 w405 w421 w437 w453] -> w365
          frame "Custom FOV" {
            n180 = local read "Xstart"() -> (w378:i32)
            n181 = local read "Xend"() -> (w377:i32)
            n182 = local read "Ystart"() -> (w375:i32)
            n183 = local read "Yend"() -> (w376:i32)
            n184 = Subtract(x=w376, y=w375) -> (x-y=w387:i32)
            n185 = Subtract(x=w377, y=w378) -> (x-y=w388:i32)
            n186 = local read "Xbin"() -> (w380:i32)
            n187 = local read "Ybin"() -> (w379:i32)
            n188 = Increment(x=w387) -> (x+1=w386:i32)
            n189 = Increment(x=w388) -> (x+1=w385:i32)
            n190 = Divide(x=w386, y=w379) -> (x/y=w382:dbl)
            n191 = Divide(x=w385, y=w380) -> (x/y=w384:dbl)
            n192 = To Long Integer(number=w382) -> (32bit integer=w381:i32)
            n193 = To Long Integer(number=w384) -> (32bit integer=w383:i32)
          }
          frame "FOV: 768x768" {
            w389 = 768
            w399 = 2.0
            w404 = 1
            n194 = Subtract(x=w403, y=w389) -> (x-y=w401:i32)
            n195 = Subtract(x=w402, y=w389) -> (x-y=w400:i32)
            n196 = Divide(x=w400, y=w399) -> (x/y=w397:dbl)
            n197 = Divide(x=w401, y=w399) -> (x/y=w398:dbl)
            n198 = Decrement(x=w389) -> (x-1=w392:i32)
            n199 = Round To Nearest(number=w398) -> (nearest integer value=w396:dbl)
            n200 = Round To Nearest(number=w397) -> (nearest integer value=w395:dbl)
            n201 = To Long Integer(number=w396) -> (32bit integer=w394:i32)
            n202 = To Long Integer(number=w395) -> (32bit integer=w393:i32)
            n203 = Add(x=w392, y=w394) -> (x+y=w391:i32)
            n204 = Add(x=w392, y=w393) -> (x+y=w390:i32)
          }
          frame "FOV: 512x512" {
            w405 = 512
            w415 = 2.0
            w420 = 1
            n205 = Subtract(x=w419, y=w405) -> (x-y=w417:i32)
            n206 = Subtract(x=w418, y=w405) -> (x-y=w416:i32)
            n207 = Divide(x=w416, y=w415) -> (x/y=w413:dbl)
            n208 = Divide(x=w417, y=w415) -> (x/y=w414:dbl)
            n209 = Decrement(x=w405) -> (x-1=w408:i32)
            n210 = Round To Nearest(number=w414) -> (nearest integer value=w412:dbl)
            n211 = Round To Nearest(number=w413) -> (nearest integer value=w411:dbl)
            n212 = To Long Integer(number=w412) -> (32bit integer=w410:i32)
            n213 = To Long Integer(number=w411) -> (32bit integer=w409:i32)
            n214 = Add(x=w408, y=w410) -> (x+y=w407:i32)
            n215 = Add(x=w408, y=w409) -> (x+y=w406:i32)
          }
          frame "FOV: 320x320" {
            w421 = 320
            w431 = 2.0
            w436 = 1
            n216 = Subtract(x=w435, y=w421) -> (x-y=w433:i32)
            n217 = Subtract(x=w434, y=w421) -> (x-y=w432:i32)
            n218 = Divide(x=w432, y=w431) -> (x/y=w429:dbl)
            n219 = Divide(x=w433, y=w431) -> (x/y=w430:dbl)
            n220 = Decrement(x=w421) -> (x-1=w424:i32)
            n221 = Round To Nearest(number=w430) -> (nearest integer value=w428:dbl)
            n222 = Round To Nearest(number=w429) -> (nearest integer value=w427:dbl)
            n223 = To Long Integer(number=w428) -> (32bit integer=w426:i32)
            n224 = To Long Integer(number=w427) -> (32bit integer=w425:i32)
            n225 = Add(x=w424, y=w426) -> (x+y=w423:i32)
            n226 = Add(x=w424, y=w425) -> (x+y=w422:i32)
          }
          frame "FOV: 256x256" {
            w437 = 256
            w447 = 2.0
            w452 = 1
            n227 = Subtract(x=w451, y=w437) -> (x-y=w449:i32)
            n228 = Subtract(x=w450, y=w437) -> (x-y=w448:i32)
            n229 = Divide(x=w448, y=w447) -> (x/y=w445:dbl)
            n230 = Divide(x=w449, y=w447) -> (x/y=w446:dbl)
            n231 = Decrement(x=w437) -> (x-1=w440:i32)
            n232 = Round To Nearest(number=w446) -> (nearest integer value=w444:dbl)
            n233 = Round To Nearest(number=w445) -> (nearest integer value=w443:dbl)
            n234 = To Long Integer(number=w444) -> (32bit integer=w442:i32)
            n235 = To Long Integer(number=w443) -> (32bit integer=w441:i32)
            n236 = Add(x=w440, y=w442) -> (x+y=w439:i32)
            n237 = Add(x=w440, y=w441) -> (x+y=w438:i32)
          }
          frame "Full FOV", Default {
            w455 = 1
          }
        }
        n238 = local write "FOV X Pixels"(w365) -> ()
        n239 = local write "FOV Y Pixels"(w364) -> ()
        n240 = call <userlib>:"SetImage.vi"("hbin"=w368, "vbin"=w369, "hstart"=w370, "hend"=w371, "vstart"=w367, "vend"=w366, "error in (no error)"=w363) -> ("error out"=w362:errorcluster)  [unwired: 19 in, 1 out]
        n241 = call <userlib>:"GetAcquisitionTimings.vi"("error in (no error)"=w362) -> ("exposure"=w359:sgl, "accumulate"=w358:sgl, "kinetic"=w357:sgl, "DLL error code"=w356:u32, "error out"=w361:errorcluster)  [unwired: 10 in]
        n242 = call <userlib>:"GetAcquisitionProgress.vi"("error in (no error)"=w361) -> ("error out"=w360:errorcluster, "DLL error code"=w353:u32, "series"=w354:i32, "accum"=w355:i32)  [unwired: 3 in]
        n243 = local write "Get Exposure Time"(w359) -> ()
        n244 = local write "Get Accum Time"(w358) -> ()
        n245 = local write "Get Kinetic Time"(w357) -> ()
        n246 = local write "Return from CheckTimings"(w356) -> ()
        n247 = local write "Return from CheckProcess"(w353) -> ()
        n248 = local write "Get Kinetic Num"(w355) -> ()
        n249 = local write "Get Kinetic Num"(w354) -> ()
      }
      event "Start LIVE": Mouse Up {
        # "Set running mode to Live Preview"
        n250 = event-data() -> ()  [unwired: 1 in, 8 out]
        n251 = flat-sequence {
          tunnel: w458 -> [w460]
          tunnel: [w460] -> w456
          tunnel: w456 -> [w463]
          tunnel: [w461] -> w457
          frame #0 {
            n252 = local write "Running Status"(1) -> ()
          }
          frame #1 {
            w462 = u16 1  # AcquisitionMode
            # "Set Acquisition Mode: Single Scan"
            n253 = call <userlib>:"SetAcquisitionMode.vi"("error in (no error)"=w463, "mode"=w462) -> ("error out"=w461:errorcluster)  [unwired: 1 out]
          }
        }
      }
      event "Stop LIVE": Mouse Up {
        # "Stop Live Preview"
        n254 = event-data() -> ()  [unwired: 1 in, 8 out]
        n255 = flat-sequence {
          tunnel: w467 -> [w469]
          tunnel: [w469] -> w464
          tunnel: [w473] -> w466
          tunnel: w464 -> [w472]
          tunnel: [w475] -> w465
          tunnel: w466 -> [w475]
          frame #0 {
            n256 = local write "Running Status"(0) -> ()
          }
          frame #1 {
            # "Recover Acquisition Mode: As Input"
            n257 = local read "Aquisition Mode"() -> (w471:T2)
            n258 = To Unsigned Word Integer(number=w471) -> (unsigned 16bit integer=w470:u16)
            n259 = call <userlib>:"SetAcquisitionMode.vi"("error in (no error)"=w472, "mode"=w470) -> ("error out"=w473:errorcluster)  [unwired: 1 out]
          }
          frame #2 {
            n260 = local write "EMCCD Status"(FALSE) -> ()
          }
        }
      }
      event "Acquisition": Mouse Up {
        # "Set to running mode to Data Acquisition"
        n261 = event-data() -> ()  [unwired: 1 in, 8 out]
        n262 = local write "Running Status"(2) -> ()
      }
      event "Abort": Mouse Up {
        n263 = event-data() -> ()  [unwired: 1 in, 8 out]
        n264 = local write "Running Status"(0) -> ()
        n265 = call <userlib>:"AbortAcquisition.vi"("error in (no error)"=w479) -> ("error out"=w478:errorcluster)  [unwired: 1 in, 1 out]
      }
      event "Intensity Max": Value Change {
        n266 = event-data() -> ()  [unwired: 1 in, 6 out]
      }
      event "Intensity Min": Value Change {
        n267 = event-data() -> ()  [unwired: 1 in, 6 out]
      }
      event "Exit": Mouse Up {
        n268 = event-data() -> ()  [unwired: 1 in, 8 out]
      }
      event Panel Close? {
        n269 = event-data() -> ()  [unwired: 1 in, 4 out]
        n270 = event-data("Discard?"=TRUE) -> ()  [unwired: 1 in, 1 out]
      }
    }
    n271 = Wait (ms)(milliseconds to wait=u32 250) -> ()  [unwired: 1 out]
    n272 = local write "error out"(w179) -> ()
  }
  n273 = case shown="True" "Abort" {
    frame False {
    }
    frame True {
    }
  }
  n274 = case shown="True" w2 {
    tunnel: w9 -> [w488 w492]
    tunnel: [w487 w491] -> w8
    tunnel: [w486 w490] -> w7
    frame False {
      n275 = call <userlib>:"GetTemperature.vi"("error in (no error)"=w488) -> ("error out"=w487:errorcluster, "temperature"=w486:i32)  [unwired: 3 in, 2 out]
    }
    frame True {
      n276 = call "iXon_Shutdown.vi"("error in (no error)"=w492, "TurnOFFCooler"=TRUE) -> ("error out"=w491:errorcluster, "Current Temp"=w490:i32)  [unwired: 8 in]
    }
  }
  "error out" <- w8
  n277 = local write "Current Temp"(w7) -> ()
